vi "Verify User.vi"(8 "ROLE":string(combo), 9 "OLD PASSWORD in":string, 10 "Authenticated Data":string[][](array[string]), 11 "User Cred":T1) -> (1 "Administator?":bool, 2 "OLD PASSWORD out":string, 3 "Password True?":bool)   [LabVIEW 2022 SP3]
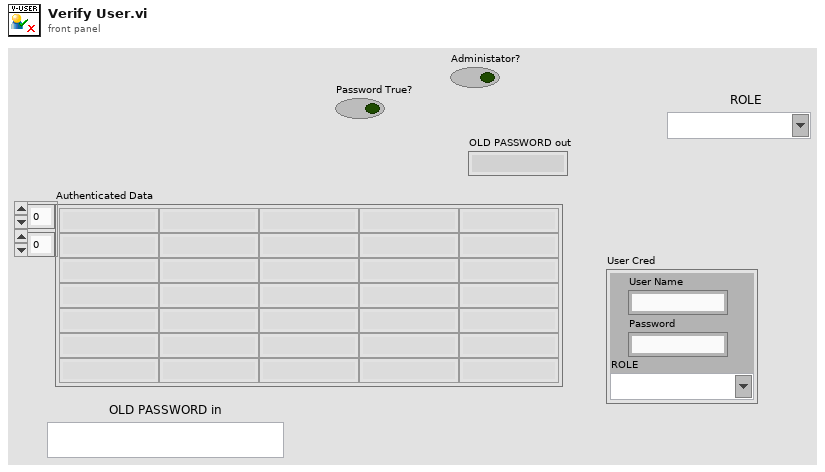
[diagram p1: front panel]
types:
  T1 = cluster{"User Name":string, "Password":string, "ROLE":string}
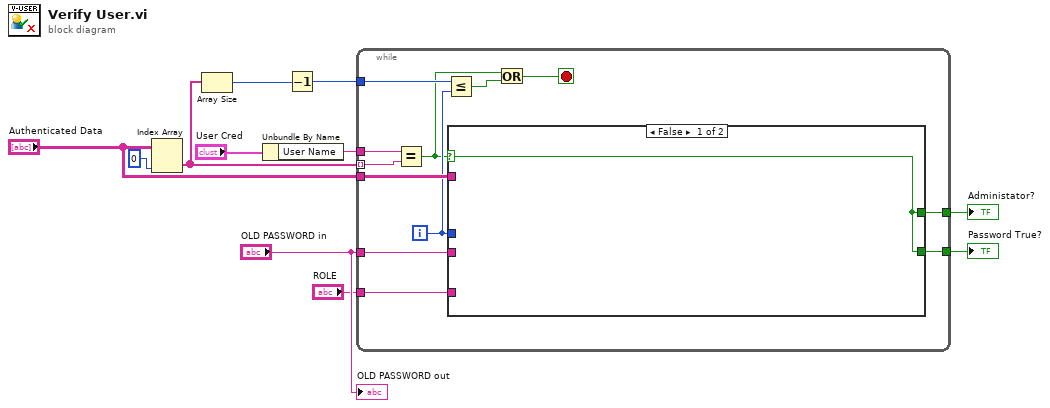
[diagram p0: block diagram]
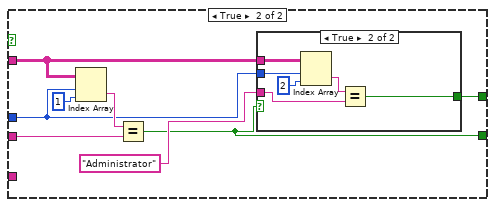
[diagram p2: hidden frame]
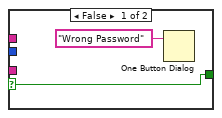
[diagram p3: hidden frame]
diagram:
  n1 = Index Array(array="Authenticated Data", index (col)=0 ("disabled index (col)")) -> (element=w6:string[])  [unwired: 1 in]
  n2 = Array Size(array=w6) -> (size(s)=w7:i32)
  n3 = Unbundle By Name("User Cred") -> ("User Name"=w5:string)
  n4 = Decrement(x=w7) -> (x-1=w10:i32)
  n5 = while {
    tunnel: w10 -> [w23]
    tunnel: w6 -> [w22] mode=indexing
    tunnel: "Authenticated Data" -> [w20]
    tunnel: w5 -> [w17]
    tunnel: "OLD PASSWORD in" -> [w18]
    tunnel: [w16] -> w9
    tunnel: [w13] -> w3
    tunnel: "ROLE" -> [w12]
    i -> [w19]
    stop <- w21 stop-if-true
    n6 = Equal?(x=w17, y=w22) -> (x = y?=w14:bool)
    n7 = Less Or Equal?(x=w23, y=w19) -> (x <= y?=w15:bool)
    n8 = case shown="False" w14 {
      selector: w14 -> [w24 _]
      tunnel: w20 -> [_ w29]
      tunnel: w19 -> [_ w28]
      tunnel: [w24 w25] -> w16
      tunnel: w18 -> [_ w31]
      tunnel: [w24 w27] -> w13
      tunnel: w12 -> [_ _]
      frame False {
      }
      frame True {
        n9 = Index Array(array=w29, index (row)=w28, index (col)=1 ("disabled index (col)")) -> (element=w30:string)
        n10 = Equal?(x=w30, y=w31) -> (x = y?=w25:bool)
        n11 = case shown="True" w25 {
          selector: w25 -> [w34 _]
          tunnel: w29 -> [_ w40]
          tunnel: w28 -> [_ w39]
          tunnel: [w34 w36] -> w27
          tunnel: "Administrator" -> [_ w35]
          frame False {
            n12 = One Button Dialog(message="Wrong Password") -> ()  [unwired: 1 in, 1 out]
          }
          frame True {
            n13 = Index Array(array=w40, index (row)=w39, index (col)=2 ("disabled index (col)")) -> (element=w37:string)
            n14 = Equal?(x=w37, y=w35) -> (x = y?=w36:bool)
          }
        }
      }
    }
    n15 = Or(x=w14, y=w15) -> (x .or. y?=w21:bool)
  }
  "Password True?" <- w9
  "Administator?" <- w3
  "OLD PASSWORD out" <- "OLD PASSWORD in"
